vi "Configure Filter Value.vi"(8 "error in (no error)":errorcluster, 9 "Filter Value for Analog to Digital Conversion ( 3 )":i32=3 min=1 max=15, 10 "Averaging Value ( 4 )":i32=4 min=0 max=16, 11 "VISA resource name":refnum<visa-resource-name>) -> (0 "error out":errorcluster, 3 "VISA resource out":refnum<visa-resource-name>)   [LabVIEW 2011, in "Ocean Server OS4000.lvlib"]
doc: "Set the average filter on roll, pitch and heading i.e number of samples to include in average.\n\nSet the digital filter value for Analog-to-Digital conversion, higher=longer filter time."
uses:
  Ocean Server OS4000.lvlib
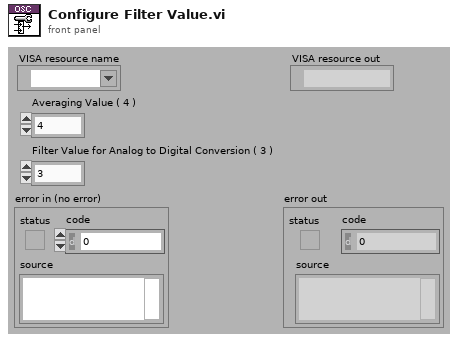
[diagram p1: front panel]
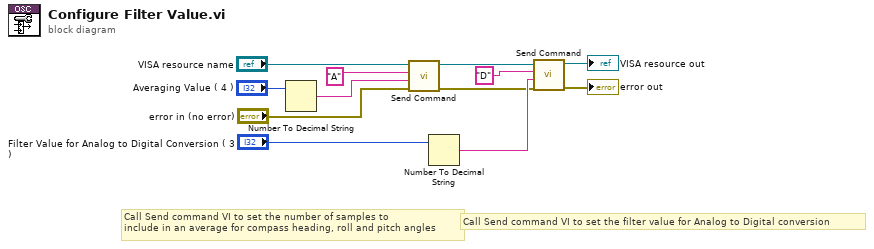
[diagram p0: block diagram]
diagram:
  # "Call Send command VI to set the filter value for Analog to Digital conversion"
  # "Call Send command VI to set the number of samples to \ninclude in an average for compass heading, roll and pitch angles"
  n1 = Number To Decimal String(number="Averaging Value ( 4 )") -> (decimal integer string=w4:string)  [unwired: 1 in]
  n2 = call "Send Command.vi"("error in (no error)"="error in (no error)", "Value"=w4, "Message"="A", "VISA resource name"="VISA resource name") -> ("error out"=w1:errorcluster, "VISA resource out"=w10:refnum<visa-resource-name>)  [unwired: 6 in]
  n3 = Number To Decimal String(number="Filter Value for Analog to Digital Conversion ( 3 )") -> (decimal integer string=w2:string)  [unwired: 1 in]
  n4 = call "Send Command.vi"("error in (no error)"=w1, "Value"=w2, "Message"="D", "VISA resource name"=w10) -> ("error out"=→"error out":errorcluster, "VISA resource out"=→"VISA resource out":refnum<visa-resource-name>)  [unwired: 6 in]
